vi "Create Listener.vi"(8 "error in":errorcluster, 11 "TCP slave in":refnum<class "TCP Server.lvclass">) -> (0 "error out":errorcluster, 3 "TCP slave out":refnum<class "TCP Server.lvclass">)   [LabVIEW 2021, in "WebSockets.lvlib" / "TCP Server.lvclass"]
doc: "Creates a new listener on the stored port, and then stores that in the class."
uses:
  TCP Server.lvclass
  D:/my_projects/projects/Algorithms/Labview/21/WebSockets/Source/WebSockets/WebSocket/WebSocket.lvclass
  WebSocket/WebSocket.lvclass/WebSocket.ctl
  Sockets/VISA TCP Socket/VISA TCP.lvclass/VISA TCP.ctl
  TCP Server.lvclass/TCP Server.ctl
  WebSocket/Read Socket.vi
  Sockets/VISA TCP Socket/VISA TCP.lvclass
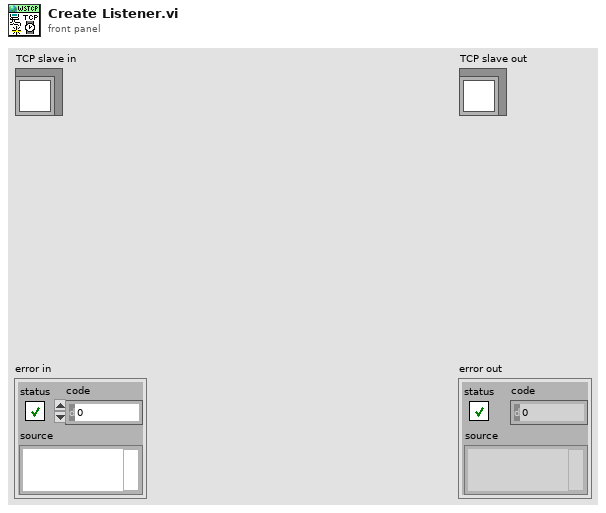
[diagram p1: front panel]
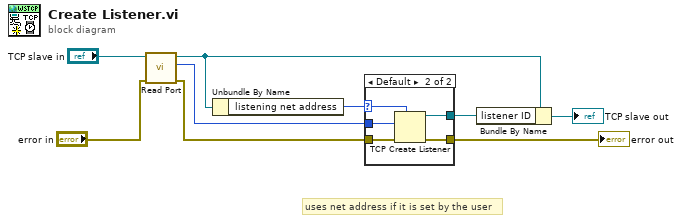
[diagram p0: block diagram]
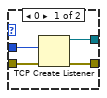
[diagram p2: hidden frame]
diagram:
  # "uses net address if it is set by the user"
  n1 = call "Read Port.vi"("error in"="error in", "TCP slave in"="TCP slave in") -> ("error out"=w4:errorcluster, "Port"=w1:u16, "TCP slave out"=w2:refnum<class "TCP Server.lvclass">)  [unwired: 7 in]
  n2 = Unbundle By Name(w2) -> ("listening net address"=w6:u32)
  n3 = case shown="Default" w6 {
    selector: w6 -> [_ w14]
    tunnel: w4 -> [w13 w18]
    tunnel: [w11 w17] -> w9
    tunnel: w1 -> [w12 w16]
    tunnel: [w10 w15] -> w7
    frame 0 {
      n4 = TCP Create Listener(8:w13, 10:w12) -> (0:w11:errorcluster, 3:w10:refnum<k5>)  [unwired: 3 in, 1 out]
    }
    frame Default {
      n5 = TCP Create Listener(7:w14, 8:w18, 10:w16) -> (0:w17:errorcluster, 3:w15:refnum<k5>)  [unwired: 2 in, 1 out]
    }
  }
  "error out" <- w9
  n6 = Bundle By Name(cluster=w2, "listener ID"=w7) -> (→"TCP slave out":refnum<class "TCP Server.lvclass">)
